vi "FA_TeamKeyValue.vi"(8 "error in":errorcluster, 10 "Array in":T1[](array[typedef])) -> (0 "error out":errorcluster, 3 "Array out":string[](array[string]))   [LabVIEW 2014, in "FA_FIRST.lvlib"]
uses:
  FA_FIRST.lvlib
  FIRST Client/source/VI Source/FC_Team Attributes.ctl
  FIRST Client/source/VI Source/FC_FIRST Client.lvlib
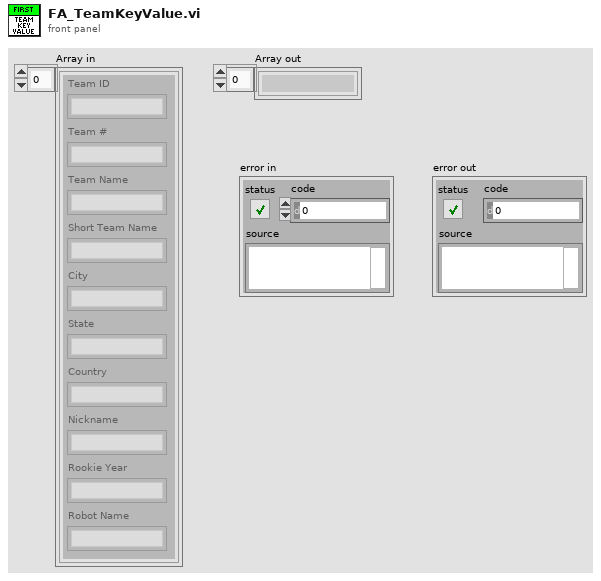
[diagram p1: front panel]
types:
  T1 = typedef "FC_FIRST Client.lvlib/FC_Team Attributes.ctl" = cluster{"Team ID":string, "Team #":string, "Team Name":string, "Short Team Name":string, "City":string, "State":string, "Country":string, "Nickname":string, "Rookie Year":string, "Robot Name":string}
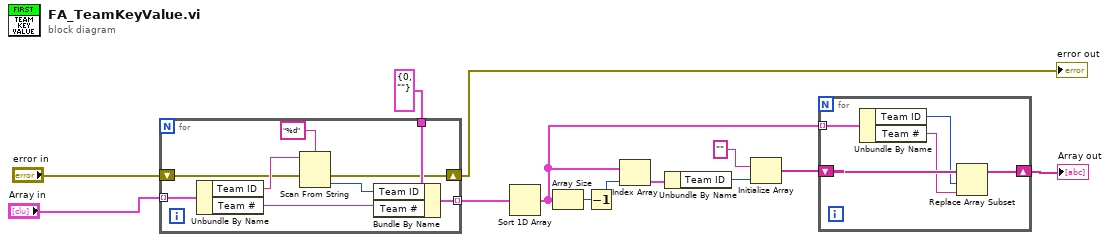
[diagram p0: block diagram]
diagram:
  n1 = for {
    tunnel: "Array in" -> [w22] mode=indexing
    tunnel: cluster{"Team ID":i32, "Team #":string} {"Team ID"=0, "Team #"=""} ("input cluster") -> [w19]
    tunnel: [w16] -> w9 mode=indexing
    shift-right: [w14] -> w1
    shift-left: "error in" -> [w15]
    n2 = Unbundle By Name(w22) -> ("Team ID"=w21:string, "Team #"=w17:string)
    n3 = Scan From String(format string="%d", input string=w21, error in=w15) -> (error out=w14:errorcluster, output 1=w18:i32)  [unwired: 2 in, 2 out]
    n4 = Bundle By Name(cluster=w19, "Team ID"=w18, "Team #"=w17) -> (w16:cluster{"Team ID":i32, "Team #":string})
  }
  "error out" <- w1
  n5 = Sort 1D Array(array=w9) -> (sorted array=w12:cluster{"Team ID":i32, "Team #":string}[])
  n6 = Array Size(array=w12) -> (size(s)=w5:i32)
  n7 = Decrement(x=w5) -> (x-1=w6:i32)
  n8 = Index Array(array=w12, index=w6) -> (element=w7:cluster{"Team ID":i32, "Team #":string})
  n9 = Unbundle By Name(w7) -> ("Team ID"=w10:i32)
  n10 = Initialize Array("", w10) -> (w2:string[])
  n11 = for {
    shift-right: [w26] -> w13
    shift-left: w2 -> [w27]
    tunnel: w12 -> [w25] mode=indexing
    n12 = Unbundle By Name(w25) -> ("Team ID"=w23:i32, "Team #"=w24:string)
    n13 = Replace Array Subset(array=w27, new element=w24, index=w23) -> (w26:string[])
  }
  "Array out" <- w13
